vi "Read Project Description.vi"(8 "error in (no error)":errorcluster, 11 "Project in":refnum<class "Project.lvclass">) -> (0 "error out":errorcluster, 2 "Project Description":string, 3 "Project out":refnum<class "Project.lvclass">)   [LabVIEW 2019, in "Panther Dashboard.lvlib" / "Project.lvclass"]
uses:
  Project.lvclass
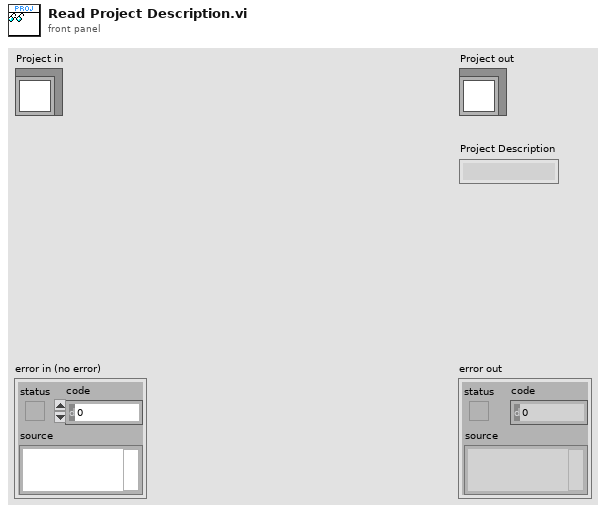
[diagram p1: front panel]
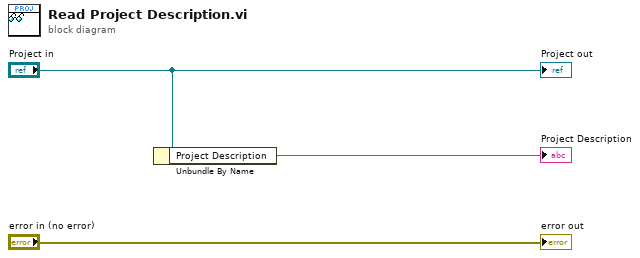
[diagram p0: block diagram]
diagram:
  n1 = Unbundle By Name("Project in") -> ("Project Description"=→"Project Description":string)
  "error out" <- "error in (no error)"
  "Project out" <- "Project in"
